vi "WriteOutputTunnels.vi"(5 "outputs":refnum<class "Tunnel.lvclass">[](array[class]), 9 "Structure in":refnum<class "Structure.lvclass">) -> (3 "Structure out":refnum<class "Structure.lvclass">)   [LabVIEW 2014, in "Raspberry Pi Compatible Compiler for LabVIEW.lvlib" / "Structure.lvclass"]
uses:
  Structure.lvclass
  Tunnel/Tunnel.lvclass
  Structure.lvclass/Structure.ctl
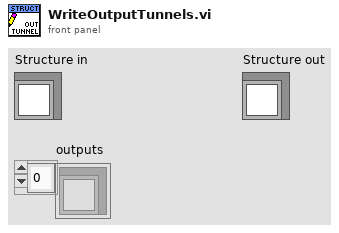
[diagram p1: front panel]
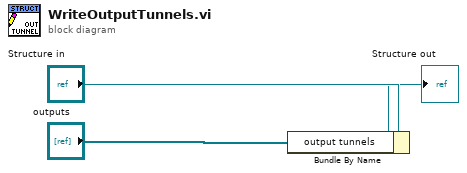
[diagram p0: block diagram]
diagram:
  n1 = Bundle By Name(cluster="Structure in", "output tunnels"="outputs") -> (→"Structure out":refnum<class "Structure.lvclass">)
